vi "SLL Fit VI window to Selected Decoration with option.vi"(6 "Object No":i32=1, 7 "Reference":enum16{"Top Left", "Bottom Right"}(ring), 8 "error in (no error)":errorcluster, 10 "border spacing":u32=2, 11 "VI Ref (calling VI)":refnum<vi>) -> (0 "error out":errorcluster, 3 "VI Ref out":refnum<vi>)   [LabVIEW 2013]
doc: "This utility will fit (resize and center) a VI (defined by the \"VI Ref\" input) about the given largest decoration in that VI. It will add a border defined by border spacing in units of pixels. If there are no decorations found in the VI it is a no-op and will not produce an error. Unfortunately, this VI can not find locked decorations (yet).\n\nUsage Caveat: If the caller VI's <B>Minimum Panel Size</B> is set to a size larger than the size of its largest decoration, this VI will give out an error.\n\nCopyright © 2006, Soliton Technologies. All rights reserved."
panel:
  in  "Case Constant\n(See Context Help)":bool
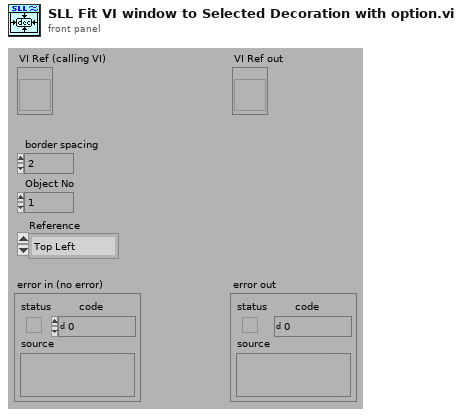
[diagram p1: front panel]
types:
  T1 = typedef "LVRectTypeDef.ctl" = cluster{"Left":i16, "Top":i16, "Right":i16, "Bottom":i16}
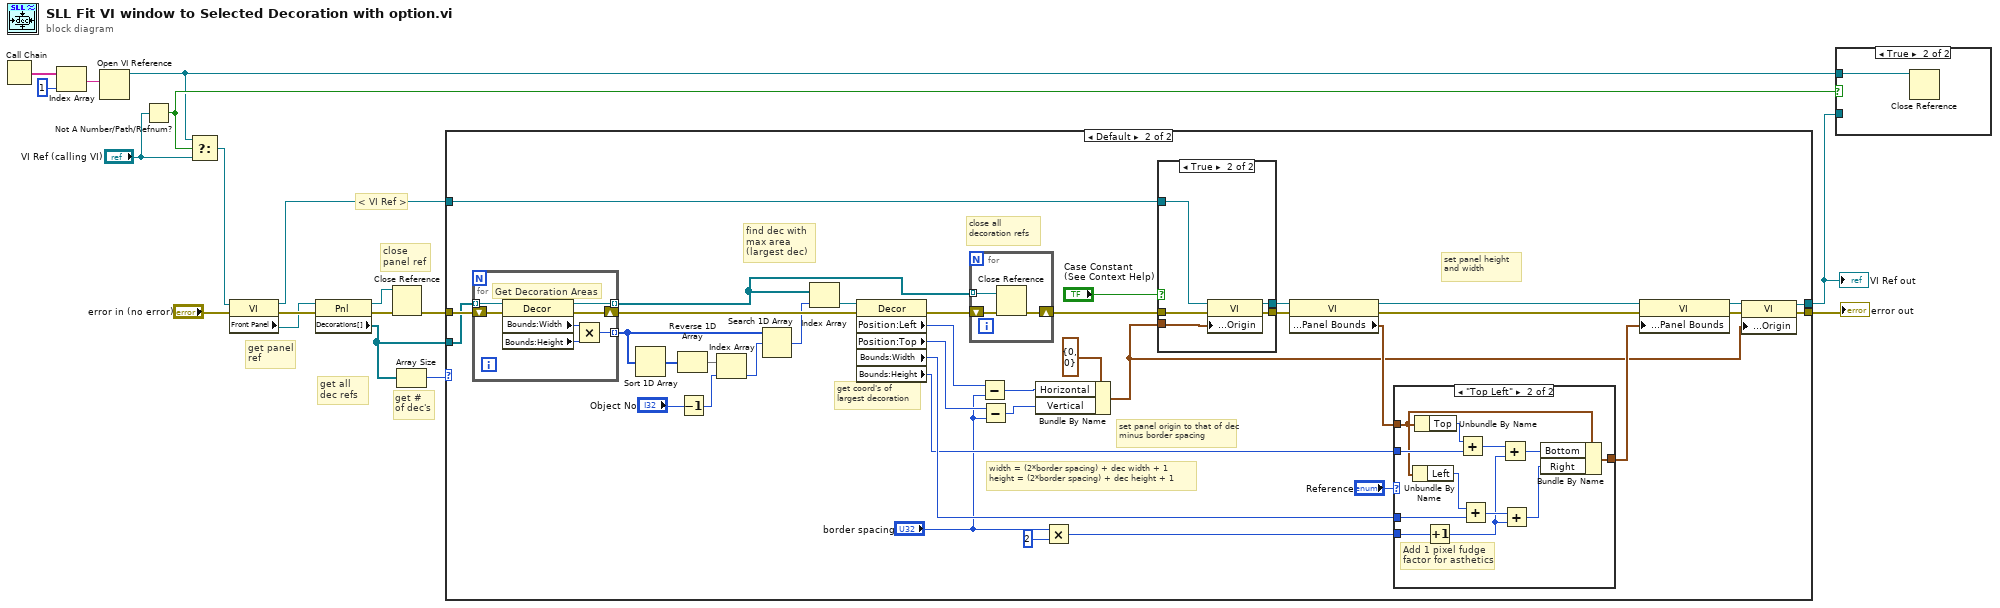
[diagram p0: block diagram]
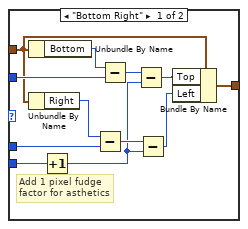
[diagram p4: hidden frame]
diagram:
  # "get # of dec's"
  # "get panel ref"
  # "get all dec refs"
  # "close panel ref"
  # "< VI Ref >"
  n1 = Call Chain() -> (call chain=w10:string[])
  n2 = Index Array(array=w10, index=1 ("Index")) -> (element=w8:string)
  n3 = Open VI Reference(vi path=w8) -> (vi reference=w3:refnum<vi>)  [unwired: 5 in, 1 out]
  n4 = Not A Number/Path/Refnum?(number/path/refnum="VI Ref (calling VI)") -> (NaN/Path/Refnum?=w4:bool)
  n5 = Select(t=w3, s=w4, f="VI Ref (calling VI)") -> (s? t:f=w7:refnum<vi>)
  n6 = property on="Property Node" class="VI"(reference=w7, error in="error in (no error)") -> (reference out=w18:refnum<vi>, error out=w16:errorcluster, "Front Panel"=w13:refnum<vi>)
  n7 = property on="Property Node" class="Pnl"(reference=w13, error in=w16) -> (reference out=w17:refnum<vi>, error out=w15:errorcluster, "Decorations[]"=w2:refnum<vi>[])
  n8 = Close Reference(reference=w17, error in (no error)=w15) -> (error out=w12:errorcluster)
  n9 = Array Size(array=w2) -> (size(s)=w1:i32)
  n10 = case shown="Default" w1 {
    tunnel: w18 -> [w20 w56]
    tunnel: w12 -> [w19 w46]
    tunnel: [w19 w23] -> w11
    tunnel: [w20 w22] -> w5
    tunnel: w2 -> [_ w35]
    frame 0 {
      # "do nothing if no decorations"
    }
    frame Default {
      # "width = (2*border spacing) + dec width + 1\nheight = (2*border spacing) + dec height + 1"
      # "set panel height and width"
      # "set panel origin to that of dec minus border spacing"
      # "close all  decoration refs"
      # "get coord's of largest decoration"
      # "find dec with max area (largest dec)"
      n11 = for {
        tunnel: w35 -> [w96] mode=indexing
        tunnel: [w93] -> w30 mode=indexing
        shift-right: [w91] -> w43
        shift-left: w46 -> [w92]
        tunnel: [w90] -> w45 mode=indexing
        # "Get Decoration Areas"
        n12 = property class="Decor"(reference=w96, error in=w92) -> (reference out=w90:refnum<vi>, error out=w91:errorcluster, "Bounds:Width"=w95:u32, "Bounds:Height"=w94:u32)
        n13 = Multiply(x=w95, y=w94) -> (x*y=w93:u32)
      }
      n14 = Sort 1D Array(array=w30) -> (sorted array=w34:u32[])
      n15 = Reverse 1D Array(array=w34) -> (reversed array=w33:u32[])
      n16 = Decrement(x="Object No") -> (x-1=w31:i32)
      n17 = Index Array(array=w33, index=w31) -> (element=w28:u32)
      n18 = Search 1D Array(1D array=w30, element=w28) -> (index of element=w29:i32)  [unwired: 1 in]
      n19 = Index Array(array=w45, index=w29) -> (element=w44:refnum<vi>)
      n20 = property class="Decor"(reference=w44, error in=w43) -> (error out=w42:errorcluster, "Position:Left"=w48:i32, "Position:Top"=w51:i32, "Bounds:Width"=w54:u32, "Bounds:Height"=w53:u32)  [unwired: 1 out]
      n21 = for {
        tunnel: w45 -> [w99] mode=indexing
        shift-right: [w97] -> w38
        shift-left: w42 -> [w98]
        n22 = Close Reference(reference=w99, error in (no error)=w98) -> (error out=w97:errorcluster)
      }
      n23 = Subtract(x=w48, y="border spacing") -> (x-y=w49:u32)
      n24 = Subtract(x=w51, y="border spacing") -> (x-y=w50:u32)
      n25 = Bundle By Name(cluster=cluster{"Horizontal":i16, "Vertical":i16} {"Horizontal"=0, "Vertical"=0} ("Front Panel Window:Origin"), "Horizontal"=w49, "Vertical"=w50) -> (w21:cluster{"Horizontal":i16, "Vertical":i16})
      n26 = Multiply(x="border spacing", y=u32 2) -> (x*y=w40:u32)
      n27 = case shown="True" "Case Constant\n(See Context Help)" {
        tunnel: [w60 w65] -> w57
        tunnel: w56 -> [w60 w64]
        tunnel: w21 -> [_ w63]
        tunnel: w38 -> [w59 w62]
        tunnel: [w59 w61] -> w37
        frame False {
        }
        frame True {
          n28 = property on="Property Node" class="VI"(reference=w64, error in=w62, "Front Panel Window:Origin"=w63) -> (reference out=w65:refnum<vi>, error out=w61:errorcluster)
        }
      }
      n29 = property on="Property Node" class="VI"(reference=w57, error in=w37) -> (reference out=w58:refnum<vi>, error out=w36:errorcluster, "Front Panel Window:Panel Bounds"=w52:T1)
      n30 = case shown="\"Top Left\"" "Reference" {
        tunnel: [w73 w85] -> w55
        tunnel: w54 -> [w72 w84]
        tunnel: w53 -> [w70 w82]
        tunnel: w52 -> [w68 w80]
        tunnel: w40 -> [w67 w79]
        frame "Bottom Right" {
          # "Add 1 pixel fudge factor for asthetics"
          n31 = Unbundle By Name(w68) -> ("Bottom"=w69:i16)
          n32 = Unbundle By Name(w68) -> ("Right"=w71:i16)
          n33 = Increment(x=w67) -> (x+1=w66:u32)
          n34 = Subtract(x=w71, y=w72) -> (x-y=w74:u32)
          n35 = Subtract(x=w69, y=w70) -> (x-y=w76:u32)
          n36 = Subtract(x=w76, y=w66) -> (x-y=w77:u32)
          n37 = Subtract(x=w74, y=w66) -> (x-y=w75:u32)
          n38 = Bundle By Name(cluster=w68, "Top"=w77, "Left"=w75) -> (w73:T1)
        }
        frame "Top Left" {
          # "Add 1 pixel fudge factor for asthetics"
          n39 = Unbundle By Name(w80) -> ("Left"=w83:i16)
          n40 = Unbundle By Name(w80) -> ("Top"=w81:i16)
          n41 = Increment(x=w79) -> (x+1=w78:u32)
          n42 = Add(x=w81, y=w82) -> (x+y=w88:u32)
          n43 = Add(x=w83, y=w84) -> (x+y=w86:u32)
          n44 = Add(x=w88, y=w78) -> (x+y=w89:u32)
          n45 = Add(x=w86, y=w78) -> (x+y=w87:u32)
          n46 = Bundle By Name(cluster=w80, "Bottom"=w89, "Right"=w87) -> (w85:T1)
        }
      }
      n47 = property on="Property Node" class="VI"(reference=w58, error in=w36, "Front Panel Window:Panel Bounds"=w55) -> (reference out=w25:refnum<vi>, error out=w24:errorcluster)
      n48 = property on="Property Node" class="VI"(reference=w25, error in=w24, "Front Panel Window:Origin"=w21) -> (reference out=w22:refnum<vi>, error out=w23:errorcluster)
    }
  }
  "error out" <- w11
  "VI Ref out" <- w5
  n49 = case shown="True" w4 {
    tunnel: w5 -> [_ _]
    tunnel: w3 -> [_ w100]
    frame False {
    }
    frame True {
      n50 = Close Reference(reference=w100) -> ()  [unwired: 1 in, 1 out]
    }
  }
